vi "SendBotSpeakCmd.vi"(3 "Termination":string="\r\n", 4 "command":string="PING", 5 "Last Bot":T1={"Address"="", "Reply EOF"="", "Hardware"="", "Retries"=0, "Timeout"=3000, "Open?"=FALSE}) -> (0 "response":string="169.254.32.85", 2 "Bot Settings out":T1)   [LabVIEW 2012]
uses:
  <userlib>/BotSpeak/VIs/Direct/BotSpeak_Control.ctl
  <userlib>/BotSpeak/VIs/SubVIs/BotSpeak_Globals.vi
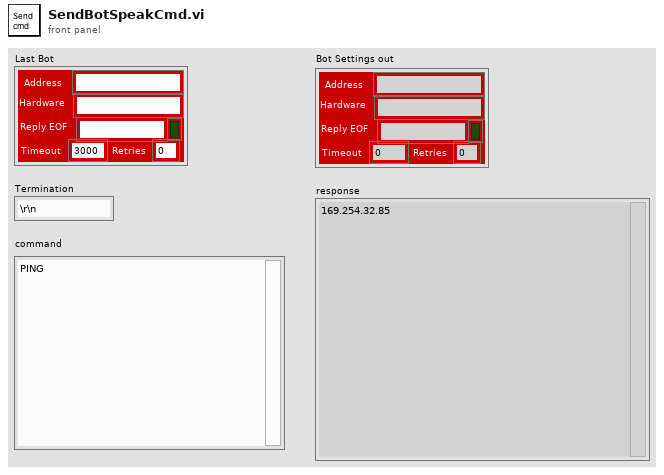
[diagram p1: front panel]
types:
  T1 = typedef "BotSpeak_Control.ctl" = cluster{"Address":string, "Reply EOF":string, "Hardware":string, "Retries":i8, "Timeout":i32, "Open?":bool}
  T2 = cluster{"Sent":string, "reply":string, "Botspeak Script":string}[]
  T3 = cluster{"Sent":string, "Reply":string, "command":string}
  T4 = cluster{"Sent":string, "Reply":string, "command":string}[]
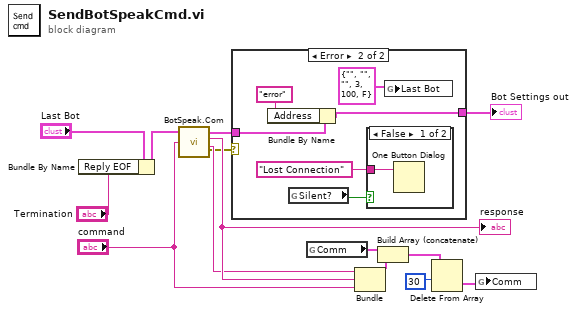
[diagram p0: block diagram]
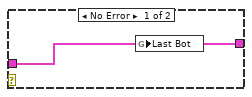
[diagram p2: hidden frame]
diagram:
  n1 = Bundle By Name(cluster="Last Bot", "Reply EOF"="Termination") -> (w14:T1)
  n2 = call <userlib>:"BotSpeak.Com.vi"("To Send"="command", "Bot Settings in"=w14) -> ("error out"=w8:errorcluster, "Sent"=w9:string, "Reply"=w10:string, "Bot Settings out"=w2:T1)  [unwired: 1 in]
  "response" <- w10
  n3 = case shown="Error" w8 {
    tunnel: [w15 w17] -> w3
    tunnel: w2 -> [w15 w21]
    frame No Error {
      n4 = global write "BotSpeak_Globals.vi" "Last Bot"(w15) -> ()
    }
    frame Error {
      n5 = Bundle By Name(cluster=w21, "Address"="error" ("Bot Settings.Address")) -> (w17:T1)
      n6 = global read "BotSpeak_Globals.vi" "Silent?"() -> (w19:bool)
      n7 = case shown="False" w19 {
        tunnel: "Lost Connection" -> [w22 _]
        frame False {
          n8 = One Button Dialog(message=w22) -> ()  [unwired: 1 in, 1 out]
        }
        frame True {
        }
      }
      n9 = global write "BotSpeak_Globals.vi" "Last Bot"(T1 {"Address"="", "Reply EOF"="", "Hardware"="", "Retries"=3, "Timeout"=100, "Open?"=FALSE} ("Last Bot")) -> ()
    }
  }
  "Bot Settings out" <- w3
  n10 = global read "BotSpeak_Globals.vi" "Comm"() -> (w7:T2)
  n11 = Bundle("Sent"=w9, "Reply"=w10, "command"="command") -> (w12:T3)  [unwired: 1 in]
  n12 = Build Array (concatenate)(w7, w12) -> (w6:T4)
  n13 = Delete From Array(array=w6, length=30) -> (deleted portion=w5:T4)  [unwired: 1 in, 1 out]
  n14 = global write "BotSpeak_Globals.vi" "Comm"(w5) -> ()
